vi "Check System Channels.vi"(8 "error in":errorcluster, 9 "Target Information in":T1, 10 "tdms file in":refnum<k34>, 11 "Telemetry System Tests in":refnum<class "Telemetry System Tests.lvclass">=refnum) -> (0 "error out":errorcluster, 1 "Target Information out":T1, 2 "tdms file out":refnum<k34>, 3 "Telemetry System Tests out":refnum<class "Telemetry System Tests.lvclass">)   [LabVIEW 2026, in "Telemetry System Tests.lvclass"]
uses:
  Telemetry System Tests.lvclass
  Source/Shared/Constants.vi
  Source/Shared/Telemetry Shared.lvlib
  <vilib>/NI/VeriStand Custom Device Testing Tools/VeriStandTestUtilities/ChassisInformation.ctl
  <vilib>/NI/VeriStand Custom Device Testing Tools/VeriStandTestUtilities/VeriStandTestUtilities.lvlib
  <vilib>/NI/VeriStand Custom Device Testing Tools/VeriStandTestUtilities/TargetInformation.ctl
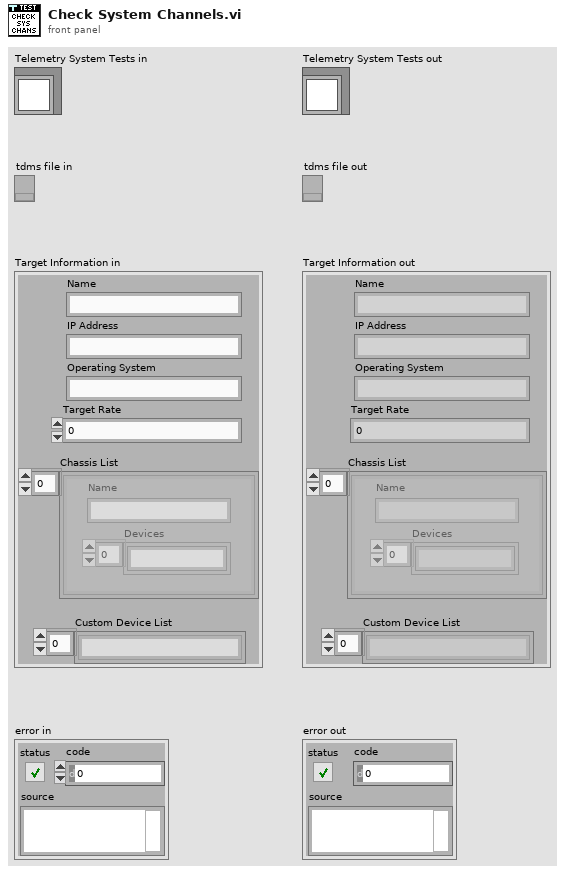
[diagram p1: front panel]
types:
  T1 = typedef "VeriStandTestUtilities.lvlib/TargetInformation.ctl" = cluster{"Name":string, "IP Address":string, "Operating System":string, "Target Rate":dbl, "Chassis List":T2[], "Custom Device List":string[]}
  T2 = typedef "VeriStandTestUtilities.lvlib/ChassisInformation.ctl" = cluster{"Name":string, "Devices":string[]}
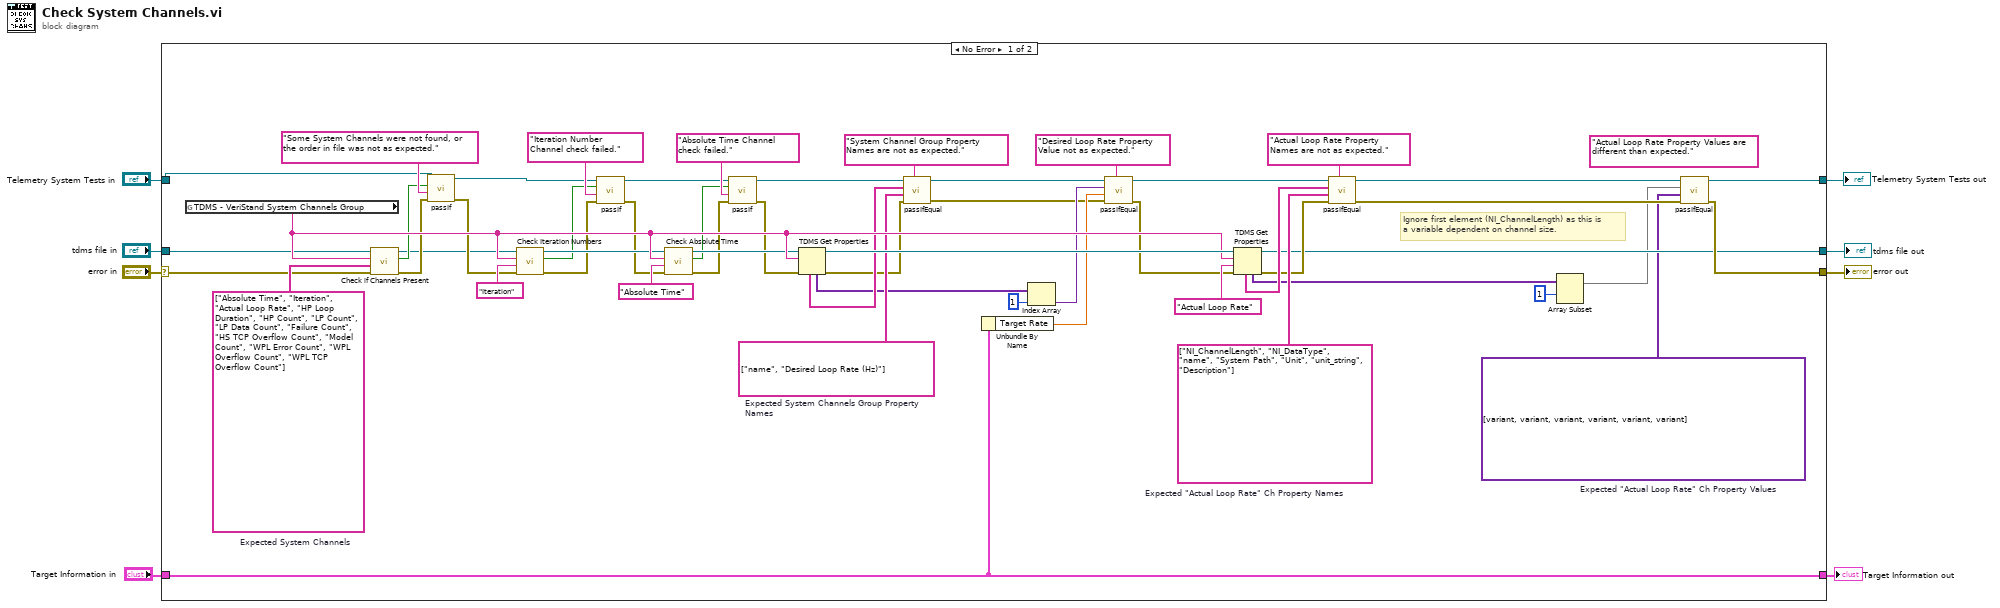
[diagram p0: block diagram]
diagram:
  n1 = case shown="No Error" "error in" {
    selector: "error in" -> [w23 w66]
    tunnel: [w61 w66] -> w8
    tunnel: [w58 w64] -> w7
    tunnel: [w53 w65] -> w6
    tunnel: "Telemetry System Tests in" -> [w27 w64]
    tunnel: "tdms file in" -> [w24 w65]
    tunnel: "Target Information in" -> [w18 w63]
    tunnel: [w18 w63] -> w1
    frame No Error {
      w9 = variant[] [variant(u16 10), variant(string "Actual Loop Rate"), variant(string "Targets/Controller/System Channels/Actual Loop Rate"), variant(string "Hz"), variant(string "Hz"), variant(string "The execution rate of the Primary Control Loop")]  # Expected "Actual Loop Rate" Ch Property Values
      (unwired) "Actual Loop Rate Property Values are different than expected." ("custom report message (\"\")")
      w59 = string[] ["NI_ChannelLength", "NI_DataType", "name", "System Path", "Unit", "unit_string", "Description"]  # Expected "Actual Loop Rate" Ch Property Names
      w50 = string[] ["name", "Desired Loop Rate (Hz)"]  # Expected System Channels Group Property Names
      w43 = string[] ["Absolute Time", "Iteration", "Actual Loop Rate", "HP Loop Duration", "HP Count", "LP Count", "LP Data Count", "Failure Count", "HS TCP Overflow Count", "Model Count", "WPL Error Count", "WPL Overflow Count", "WPL TCP Overflow Count"]  # Expected System Channels
      # "Ignore first element (NI_ChannelLength) as this is a variable dependent on channel size."
      n2 = global read "Constants.vi" "TDMS - VeriStand System Channels Group"() -> (w51:string)
      n3 = call "Check if Channels Present.vi"("error in (no error)"=w23, "Channel Names"=w43, "Group name"=w51, "Refnum in"=w24) -> ("error out"=w29:errorcluster, "Passed ?"=w31:bool, "Refnum out"=w25:refnum<k34>)  [unwired: 5 in]
      n4 = call-dynamic "passIf.vi"("error in (no error)"=w29, "message (\"\")"="Some System Channels were not found, or the order in file was not as expected." ("message (\"\")"), "pass"=w31, "TestCase in"=w27) -> ("error out"=w30:errorcluster, "TestCase out"=w28:refnum<class "Telemetry System Tests.lvclass">)  [unwired: 6 in]
      n5 = call "Check Iteration Numbers.vi"("error in (no error)"=w30, "Channel Name"="Iteration", "Group Name"=w51, "Refnum in"=w25) -> ("error out"=w33:errorcluster, "Passed ?"=w26:bool, "Refnum out"=w36:refnum<k34>)  [unwired: 5 in]
      n6 = call-dynamic "passIf.vi"("error in (no error)"=w33, "message (\"\")"="Iteration Number Channel check failed." ("message (\"\")"), "pass"=w26, "TestCase in"=w28) -> ("error out"=w35:errorcluster, "TestCase out"=w37:refnum<class "Telemetry System Tests.lvclass">)  [unwired: 6 in]
      n7 = call "Check Absolute Time.vi"("error in (no error)"=w35, "Channel Name"="Absolute Time", "Group Name"=w51, "Refnum in"=w36) -> ("error out"=w39:errorcluster, "Passed ?"=w38:bool, "Refnum out"=w45:refnum<k34>)  [unwired: 4 in, 1 out]
      n8 = call-dynamic "passIf.vi"("error in (no error)"=w39, "message (\"\")"="Absolute Time Channel check failed." ("message (\"\")"), "pass"=w38, "TestCase in"=w37) -> ("error out"=w44:errorcluster, "TestCase out"=w46:refnum<class "Telemetry System Tests.lvclass">)  [unwired: 6 in]
      n9 = TDMS Get Properties(8:w44, 10:w51, 11:w45) -> (0:w47:errorcluster, 3:w52:refnum<k34>, 4:w17:variant[], 6:w49:string[])  [unwired: 3 in, 2 out]
      n10 = call-dynamic "passIfEqual.vi"("custom report message (\"\")"="System Channel Group Property Names are not as expected." ("custom report message (\"\")"), "error in (no error)"=w47, "y"=w50, "x"=w49, "TestCase in"=w46) -> ("error out"=w13:errorcluster, "TestCase out"=w20:refnum<class "Telemetry System Tests.lvclass">)  [unwired: 5 in]
      n11 = Unbundle By Name(w18) -> ("Target Rate"=w14:dbl)
      n12 = Index Array(array=w17, index=1) -> (element=w15:variant)
      n13 = call-dynamic "passIfEqual.vi"("custom report message (\"\")"="Desired Loop Rate Property Value not as expected." ("custom report message (\"\")"), "error in (no error)"=w13, "y"=w14, "x"=w15, "TestCase in"=w20) -> ("error out"=w12:errorcluster, "TestCase out"=w19:refnum<class "Telemetry System Tests.lvclass">)  [unwired: 5 in]
      n14 = TDMS Get Properties(8:w12, 9:"Actual Loop Rate" ("channel name"), 10:w51, 11:w52) -> (0:w56:errorcluster, 3:w53:refnum<k34>, 4:w22:variant[], 6:w62:string[])  [unwired: 2 in, 2 out]
      n15 = call-dynamic "passIfEqual.vi"("custom report message (\"\")"="Actual Loop Rate Property Names are not as expected." ("custom report message (\"\")"), "error in (no error)"=w56, "y"=w59, "x"=w62, "TestCase in"=w19) -> ("error out"=w60:errorcluster, "TestCase out"=w57:refnum<class "Telemetry System Tests.lvclass">)  [unwired: 5 in]
      n16 = Array Subset(array=w22, index=1) -> (w10:variant[])  [unwired: 1 in]
      n17 = call-dynamic "passIfEqual.vi"("error in (no error)"=w60, "y"=w9, "x"=w10, "TestCase in"=w57) -> ("error out"=w61:errorcluster, "TestCase out"=w58:refnum<class "Telemetry System Tests.lvclass">)  [unwired: 6 in]
    }
    frame Error {
    }
  }
  "error out" <- w8
  "Telemetry System Tests out" <- w7
  "tdms file out" <- w6
  "Target Information out" <- w1
